vi "ClusterRef to Label-Value-Arrays.vi"(8 "error in (no error)":errorcluster, 11 "Cluster in":refnum<vi>) -> (0 "error out":errorcluster, 3 "Labels-Values Cluster":cluster{string[], variant[]})   [LabVIEW 2023]
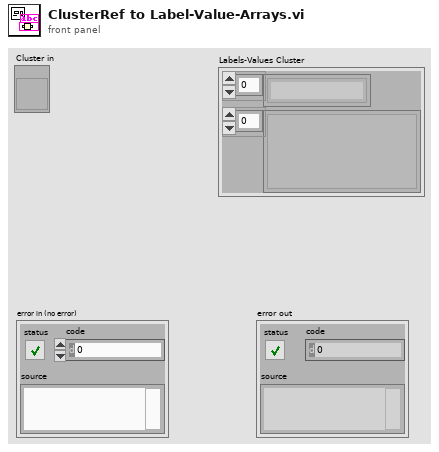
[diagram p1: front panel]
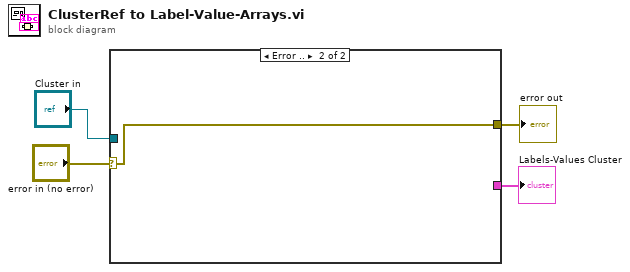
[diagram p0: block diagram]
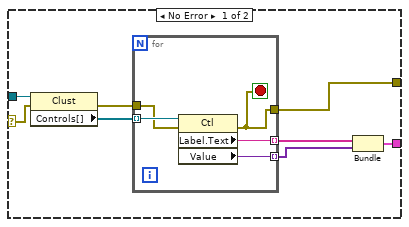
[diagram p2: hidden frame]
diagram:
  n1 = case shown="Error .." "error in (no error)" {
    selector: "error in (no error)" -> [w5 w18]
    tunnel: [w12 w18] -> w4
    tunnel: "Cluster in" -> [w9 _]
    tunnel: [w6 _] -> w2
    frame No Error {
      n2 = property class="Clust"(reference=w9, error in=w5) -> (error out=w11:errorcluster, "Controls[]"=w10:refnum<vi>[])  [unwired: 1 out]
      n3 = for {
        tunnel: w10 -> [w17] mode=indexing
        tunnel: w11 -> [w16]
        tunnel: [w15] -> w8 mode=indexing
        tunnel: [w14] -> w7 mode=indexing
        tunnel: [w13] -> w12
        stop <- w13 stop-if-true
        n4 = property class="Ctl"(reference=w17, error in=w16) -> (error out=w13:errorcluster, "Label.Text"=w15:string, "Value"=w14:variant)  [unwired: 1 out]
      }
      n5 = Bundle(w8, w7) -> (w6:cluster{string[], variant[]})  [unwired: 1 in]
    }
    frame Error {
    }
  }
  "error out" <- w4
  "Labels-Values Cluster" <- w2
